vi "Reformat malformed date-time String.vi"(10 "Date-Time String (malformed)":string) -> (2 "Date-Time String (well-formed)":string)   [LabVIEW 2009]
uses:
  <vilib>/regexp/Match Regular Expression.xnode
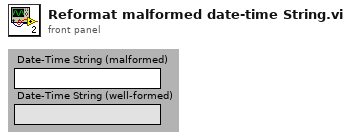
[diagram p1: front panel]
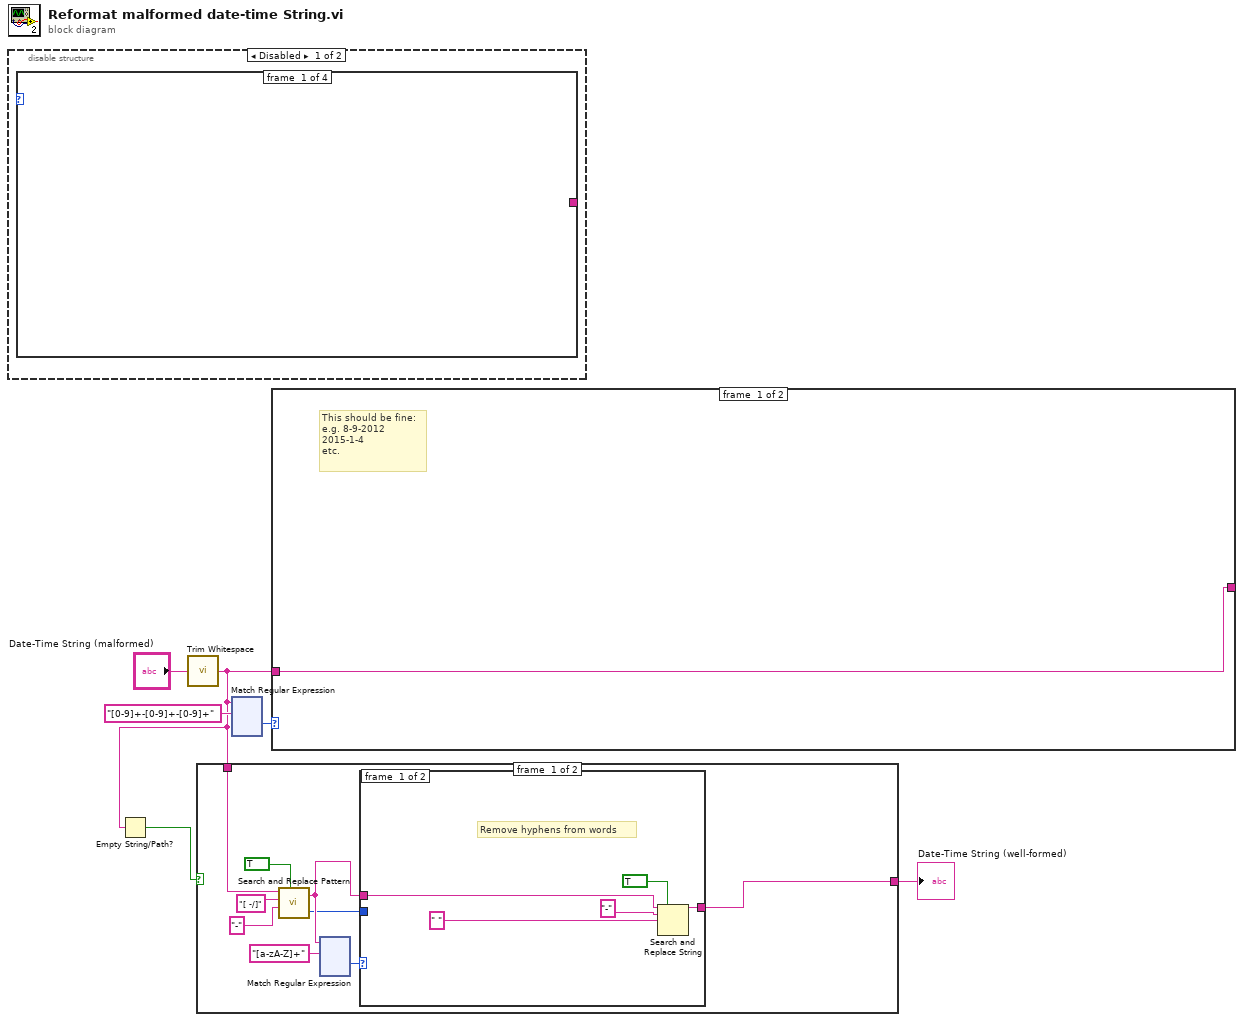
[diagram p0: block diagram]
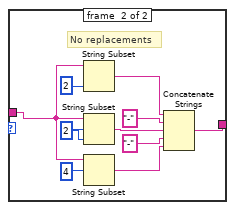
[diagram p3: hidden frame]
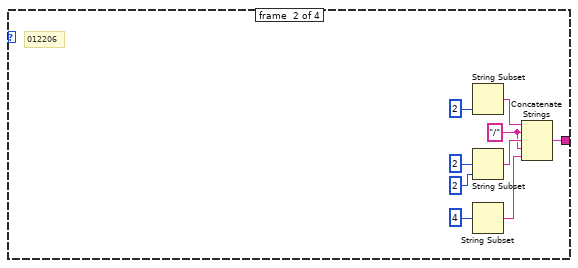
[diagram p5: hidden frame]
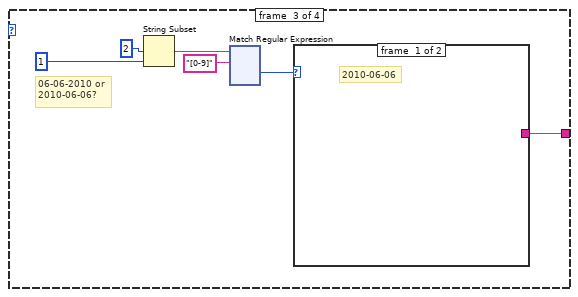
[diagram p6: hidden frame]
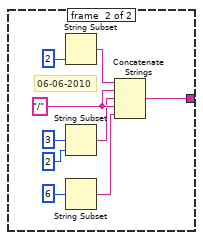
[diagram p7: hidden frame]
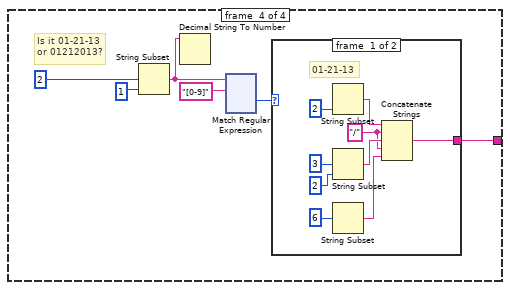
[diagram p8: hidden frame]
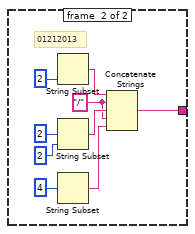
[diagram p9: hidden frame]
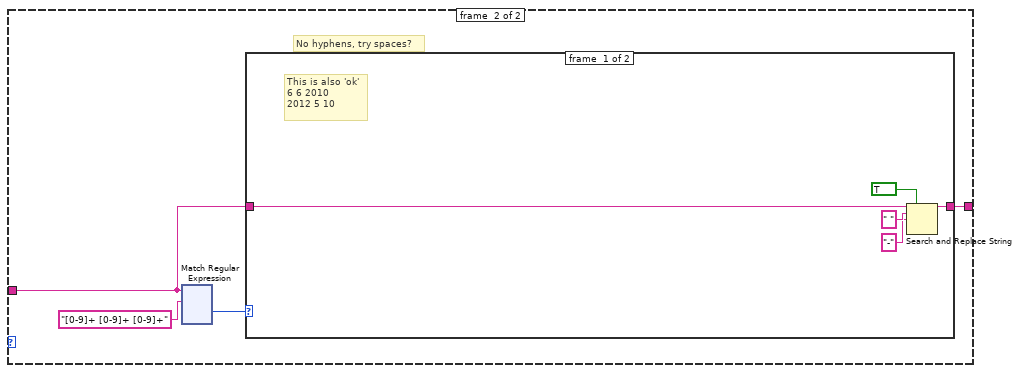
[diagram p11: hidden frame]
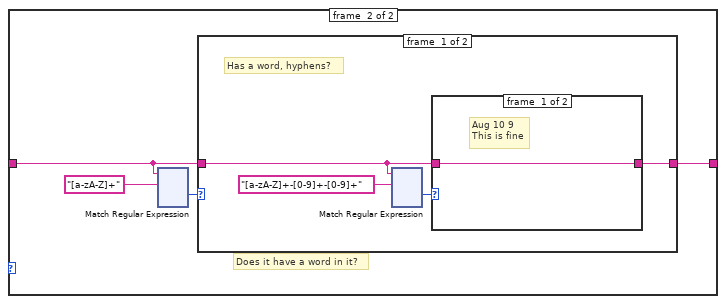
[diagram p12: hidden frame]
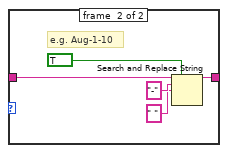
[diagram p13: hidden frame]
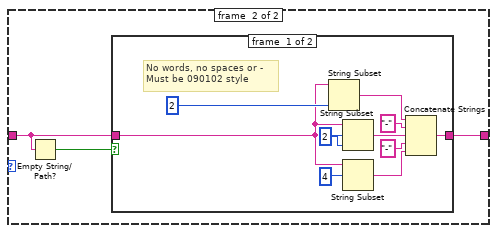
[diagram p14: hidden frame]
diagram:
  n1 = disable-structure shown="Disabled" {
    frame #0 {
      n2 = case shown="8" {
        selector: _ -> [_ _ _ _]
        tunnel: [_ w8 w19 w143] -> _
        frame #0 {
        }
        frame #1 {
          w9 = "/" ("string")
          # "012206"
          n3 = String Subset(length (rest)=2 ("length (rest)")) -> (substring=w11:string)  [unwired: 2 in]
          n4 = String Subset(offset (0)=2, length (rest)=2 ("length (rest)")) -> (substring=w10:string)  [unwired: 1 in]
          n5 = String Subset(offset (0)=4) -> (substring=w7:string)  [unwired: 2 in]
          n6 = Concatenate Strings(w11, w9, w10, w9, w7) -> (w8:string)
        }
        frame #2 {
          # "06-06-2010 or\n2010-06-06?"
          n7 = String Subset(offset (0)=2, length (rest)=1 ("length (rest)")) -> (substring=w18:string)  [unwired: 1 in]
          n8 = xnode "Match Regular Expression"("input string"=w18, "regular expression"="[0-9]") -> ("offset past match"=w16:i32)  [unwired: 4 in, 4 out]
          n9 = case shown="-1" w16 {
            tunnel: [_ w131] -> w19
            frame #0 {
              # "2010-06-06"
            }
            frame #1 {
              w136 = "/" ("string")
              # "06-06-2010"
              n10 = String Subset(length (rest)=2 ("length (rest)")) -> (substring=w129:string)  [unwired: 2 in]
              n11 = String Subset(offset (0)=3, length (rest)=2 ("length (rest)")) -> (substring=w135:string)  [unwired: 1 in]
              n12 = String Subset(offset (0)=6) -> (substring=w137:string)  [unwired: 2 in]
              n13 = Concatenate Strings(w129, w136, w135, w136, w137) -> (w131:string)
            }
          }
        }
        frame #3 {
          # "Is it 01-21-13\nor 01212013?"
          n14 = String Subset(offset (0)=2, length (rest)=1 ("length (rest)")) -> (substring=w139:string)  [unwired: 1 in]
          n15 = Decimal String To Number(string=w139) -> ()  [unwired: 2 in, 2 out]
          n16 = xnode "Match Regular Expression"("input string"=w139, "regular expression"="[0-9]") -> ("offset past match"=w138:i32)  [unwired: 4 in, 4 out]
          n17 = case shown="-1" w138 {
            tunnel: [w253 w262] -> w143
            frame #0 {
              w254 = "/" ("string")
              # "01-21-13"
              n18 = String Subset(length (rest)=2 ("length (rest)")) -> (substring=w256:string)  [unwired: 2 in]
              n19 = String Subset(offset (0)=3, length (rest)=2 ("length (rest)")) -> (substring=w255:string)  [unwired: 1 in]
              n20 = String Subset(offset (0)=6) -> (substring=w252:string)  [unwired: 2 in]
              n21 = Concatenate Strings(w256, w254, w255, w254, w252) -> (w253:string)
            }
            frame #1 {
              w263 = "/" ("string")
              # "01212013"
              n22 = String Subset(length (rest)=2 ("length (rest)")) -> (substring=w265:string)  [unwired: 2 in]
              n23 = String Subset(offset (0)=2, length (rest)=2 ("length (rest)")) -> (substring=w264:string)  [unwired: 1 in]
              n24 = String Subset(offset (0)=4) -> (substring=w261:string)  [unwired: 2 in]
              n25 = Concatenate Strings(w265, w263, w264, w263, w261) -> (w262:string)
            }
          }
        }
      }
    }
    frame #1 {
    }
  }
  n26 = call <vilib>:"Trim Whitespace.vi"("string"="Date-Time String (malformed)") -> ("trimmed string"=w3:string)  [unwired: 1 in]
  n27 = Empty String/Path?(string/path=w3) -> (empty?=w2:bool)
  n28 = case shown="False" w2 {
    tunnel: w3 -> [w273 _]
    tunnel: [w269 _] -> w1
    frame #0 {
      n29 = call <vilib>:"Search and Replace Pattern.vi"("string"=w273, "regular expression (\"\")"="[ -/]" ("regular expression (\"\")"), "replace string (\"\")"="-" ("replace string (\"\")"), "replace all? (F)"=TRUE) -> ("result string"=w272:string, "offset past match"=w271:i32)  [unwired: 1 in]
      n30 = xnode "Match Regular Expression"("input string"=w272, "regular expression"="[a-zA-Z]+") -> ("offset past match"=w276:i32)  [unwired: 4 in, 4 out]
      n31 = case shown="-1" w276 {
        tunnel: w272 -> [w388 w391]
        tunnel: [w386 w390] -> w269
        tunnel: w271 -> [_ w392]
        frame #0 {
          # "Remove hyphens from words"
          n32 = Search and Replace String(replace all?=TRUE ("replace all? (F)"), input string=w388, search string="-", replace string=" " ("replace string (\"\")")) -> (result string=w386:string)  [unwired: 4 in, 3 out]
        }
        frame #1 {
          n33 = case shown="-1" w392 {
            tunnel: w391 -> [w393 w394]
            tunnel: [w393 w395] -> w390
            frame #0 {
              # "No words, contained symbols\nall replaced."
            }
            frame #1 {
              w399 = 2 ("offset (0)")
              # "No replacements"
              n34 = String Subset(string=w394, length (rest)=2 ("length (rest)")) -> (substring=w398:string)  [unwired: 1 in]
              n35 = String Subset(string=w394, offset (0)=w399, length (rest)=w399) -> (substring=w400:string)
              n36 = String Subset(string=w394, offset (0)=4) -> (substring=w403:string)  [unwired: 1 in]
              n37 = Concatenate Strings(w398, "-" ("string"), w400, "-" ("string"), w403) -> (w395:string)
            }
          }
        }
      }
    }
    frame #1 {
    }
  }
  "Date-Time String (well-formed)" <- w1
  n38 = xnode "Match Regular Expression"("input string"=w3, "regular expression"="[0-9]+-[0-9]+-[0-9]+") -> ("offset past match"=w4:i32)  [unwired: 4 in, 4 out]
  n39 = case shown="-1" w4 {
    tunnel: w3 -> [w404 w405]
    tunnel: [w404 w406] -> _
    frame #0 {
      # "This should be fine:\ne.g. 8-9-2012\n2015-1-4\netc."
    }
    frame #1 {
      # "No hyphens, try spaces?"
      n40 = xnode "Match Regular Expression"("input string"=w405, "regular expression"="[0-9]+ [0-9]+ [0-9]+") -> ("offset past match"=w407:i32)  [unwired: 4 in, 4 out]
      n41 = case shown="-1" w407 {
        tunnel: w405 -> [w413 w415]
        tunnel: [w409 w414] -> w406
        frame #0 {
          # "This is also 'ok'\n6 6 2010\n2012 5 10"
          n42 = Search and Replace String(replace all?=TRUE ("replace all? (F)"), input string=w413, search string=" ", replace string="-" ("replace string (\"\")")) -> (result string=w409:string)  [unwired: 4 in, 3 out]
        }
        frame #1 {
          # "Does it have a word in it?"
          n43 = xnode "Match Regular Expression"("input string"=w415, "regular expression"="[a-zA-Z]+") -> ("offset past match"=w416:i32)  [unwired: 4 in, 4 out]
          n44 = case shown="-1" w416 {
            tunnel: w415 -> [w418 w536]
            tunnel: [w421 w537] -> w414
            frame #0 {
              # "Has a word, hyphens?"
              n45 = xnode "Match Regular Expression"("input string"=w418, "regular expression"="[a-zA-Z]+-[0-9]+-[0-9]+") -> ("offset past match"=w419:i32)  [unwired: 4 in, 4 out]
              n46 = case shown="Default" w419 {
                tunnel: [w422 w426] -> w421
                tunnel: w418 -> [w422 w423]
                frame #0 {
                  # "Aug 10 9\nThis is fine"
                }
                frame #1 {
                  # "e.g. Aug-1-10"
                  n47 = Search and Replace String(replace all?=TRUE ("replace all? (F)"), input string=w423, search string="-", replace string=" " ("replace string (\"\")")) -> (result string=w426:string)  [unwired: 4 in, 3 out]
                }
              }
            }
            frame #1 {
              n48 = Empty String/Path?(string/path=w536) -> (empty?=w535:bool)
              n49 = case shown="False" w535 {
                tunnel: w536 -> [w541 w548]
                tunnel: [w538 w548] -> w537
                frame #0 {
                  w544 = 2 ("offset (0)")
                  # "No words, no spaces or -\nMust be 090102 style"
                  n50 = String Subset(string=w541, length (rest)=2 ("length (rest)")) -> (substring=w545:string)  [unwired: 1 in]
                  n51 = String Subset(string=w541, offset (0)=w544, length (rest)=w544) -> (substring=w543:string)
                  n52 = String Subset(string=w541, offset (0)=4) -> (substring=w539:string)  [unwired: 1 in]
                  n53 = Concatenate Strings(w545, "-" ("string"), w543, "-" ("string"), w539) -> (w538:string)
                }
                frame #1 {
                  # "Null string"
                }
              }
            }
          }
        }
      }
    }
  }
